vi "autonomous.vi"() -> ()   [LabVIEW 2012, in "Test.lvrbt"]
uses:
  Test.lvrbt
  <vilib>/NXT/Hardware/Plugins/Tetrix DC Motor/TetrixDCMotorAddress.ctl
  <vilib>/NXT/NXTIO Xnodes/NXTIONodeSubVIs/TETRIX IO Check Battery.vi
  <vilib>/NXT/Dual Mode Library/Waits/Wait_Num(msec).vi
  <vilib>/NXT/Dual Mode Library/Waits/Wait_Num.vi
  <vilib>/NXT/NXTIO Xnodes/NXTIONodeSubVIs/TETRIX IO Move DC Motors.vi
  <vilib>/NXT/NXTIO Xnodes/NXTIONodeSubVIs/TETRIX IO Stop DC Motors.vi
  <vilib>/NXT/Subs/LVHSConnector.ctl
  <vilib>/NXT/NXTIO Xnodes/AddressXNode/NXTIOAddress.xnode
  <vilib>/NXT/NXTIO Xnodes/NXTIOXNode/NXTIO.xnode
  <vilib>/NXT/LegoClasses/BrickReference/BrickReference.lvclass
panel:
  out "Enabled":bool
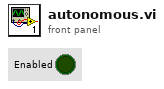
[diagram p1: front panel]
types:
  T1 = typedef "LVHSConnector.ctl" = refnum<class "BrickReference.lvclass">
  T2 = typedef "TetrixDCMotorAddress.ctl" = i32
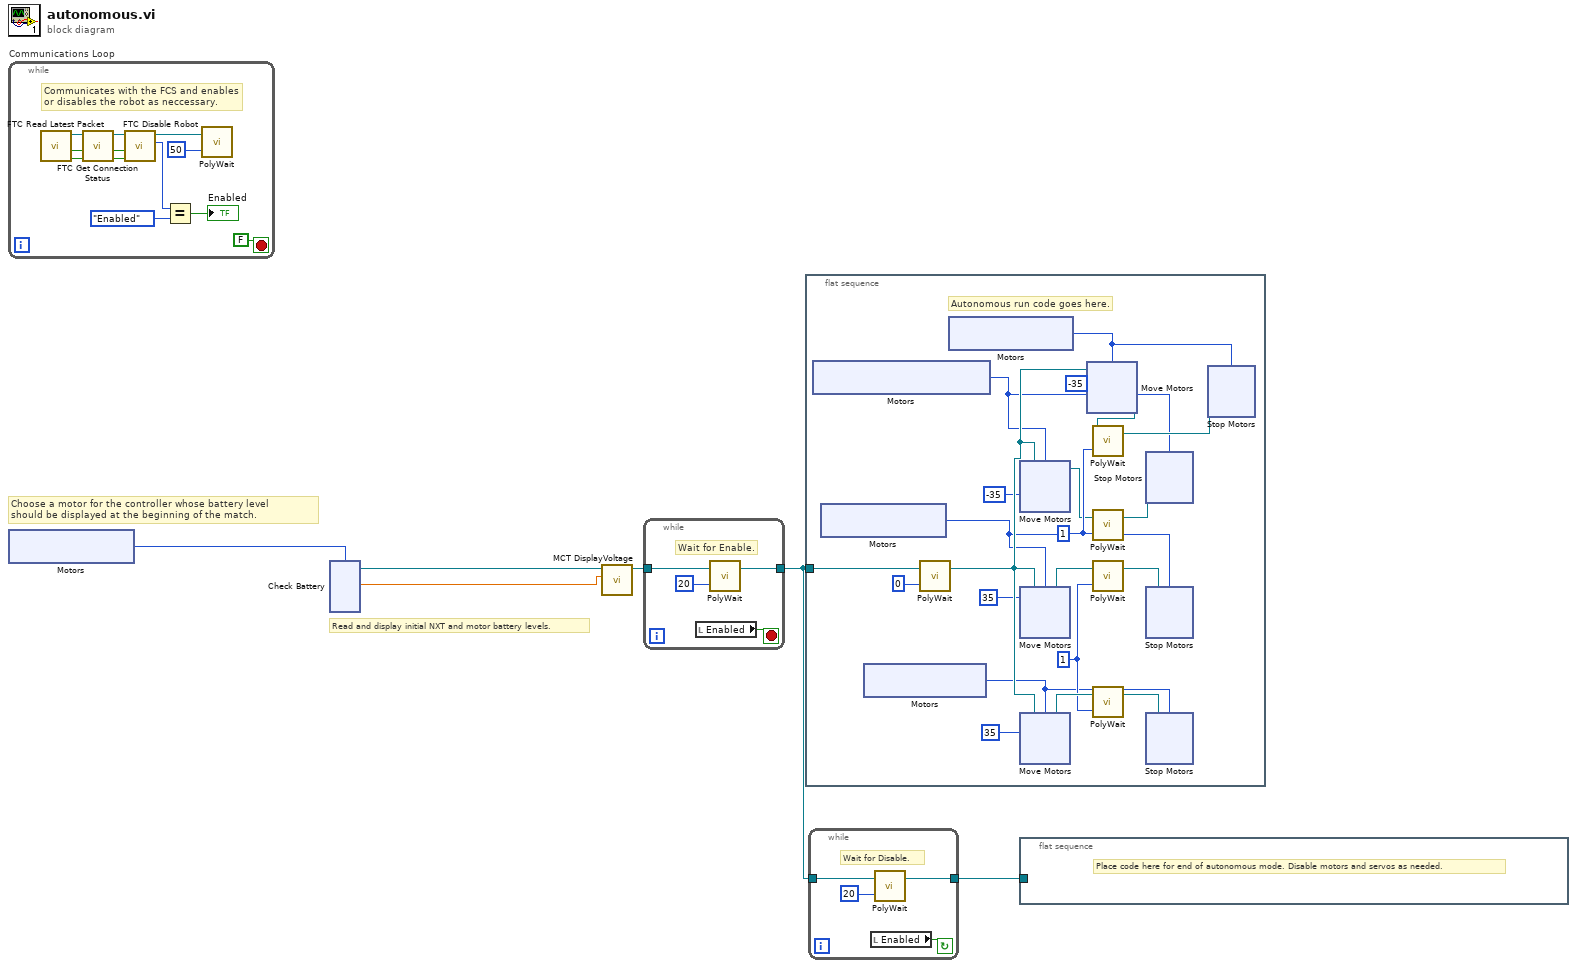
[diagram p0: block diagram]
diagram:
  # "Read and display initial NXT and motor battery levels."
  # "Choose a motor for the controller whose battery level \nshould be displayed at the beginning of the match."
  n1 = while "Communications Loop" {
    stop <- FALSE stop-if-true
    # "Communicates with the FCS and enables \nor disables the robot as neccessary."
    n2 = call <vilib>:"FTC Read Latest Packet.vi"() -> ("Packet Received?"=w16:bool, "Stopped?"=w15:bool, "NXT/EV3"=w18:T1)  [unwired: 6 in, 3 out]
    n3 = call <vilib>:"FTC Get Connection Status.vi"("Packet Received?"=w16, "Stopped?"=w15, "NXT/EV3"=w18) -> ("Online?"=w7:bool, "Stopped?"=w8:bool, "NXT/EV3"=w17:T1)  [unwired: 5 in]
    n4 = call <vilib>:"FTC Disable Robot.vi"("Online?"=w7, "Stopped?"=w8, "NXT/EV3"=w17) -> ("Enabled?"=w11:enum16{"Disabled", "Enabled"}, "NXT/EV3"=w13:T1)  [unwired: 3 in]
    n5 = Equal?(x=w11, y=enum16{"Disabled", "Enabled"}."Enabled") -> (x = y?=→"Enabled":bool)
    n6 = call-poly <vilib>:"PolyWait.vi"("Time (100 msec)"=u32 50 ("Time (msec)"), "NXT/EV3"=w13) -> ()  [unwired: 2 in, 1 out]
  }
  n7 = xnode "Motors"() -> ("Motor"=w1:T2)
  n8 = xnode "Check Battery"("Motors"=w1) -> ("Voltage 1"=w2:sgl, "NXT/EV3"=w4:T1)  [unwired: 1 in]
  n9 = call <vilib>:"MCT DisplayVoltage.vi"("Motor Voltage"=w2, "NXT/EV3"=w4) -> ("NXT/EV3"=w3:T1)  [unwired: 9 in]
  n10 = while {
    tunnel: [w20] -> w6
    tunnel: w3 -> [w19]
    stop <- w21 stop-if-true
    # "Wait for Enable."
    n11 = local read "Enabled"() -> (w21:bool)
    n12 = call-poly <vilib>:"PolyWait.vi"("Time (100 msec)"=u32 20 ("Time (msec)"), "NXT/EV3"=w19) -> ("NXT/EV3"=w20:T1)  [unwired: 2 in]
  }
  n13 = flat-sequence {
    tunnel: w6 -> [w42]
    frame #0 {
      w36 = 1
      w37 = 1
      # "Autonomous run code goes here."
      n14 = xnode "Motors"() -> ("Motor"=w29:T2)
      n15 = xnode ("Motors")() -> ("Motor"=w28:T2)
      n16 = xnode "Motors"() -> ("Motor"=w27:T2)
      n17 = call-poly <vilib>:"PolyWait.vi"("Time (1 sec)"=0, "NXT/EV3"=w42) -> ("NXT/EV3"=w31:T1)  [unwired: 2 in]
      n18 = xnode "Motors"() -> ("Motor"=w30:T2)
      n19 = xnode "Move Motors"("Power/Speed 1"=-35, "Motors"=w29, "NXT/EV3"=w31) -> ("NXT/EV3"=w35:T1)
      n20 = xnode ("Move Motors")("Power/Speed 1"=35, "Motors"=w28, "NXT/EV3"=w31) -> ("NXT/EV3"=w41:T1)
      n21 = xnode "Move Motors"("Power/Speed 1"=35, "Motors"=w27, "NXT/EV3"=w31) -> ("NXT/EV3"=w40:T1)
      n22 = xnode "Move Motors"("Power/Speed 1"=-35, "Motors"=w30, "NXT/EV3"=w31) -> ("NXT/EV3"=w32:T1)
      n23 = call-poly <vilib>:"PolyWait.vi"("Time (1 sec)"=w37, "NXT/EV3"=w32) -> ("NXT/EV3"=w33:T1)  [unwired: 2 in]
      n24 = call-poly <vilib>:"PolyWait.vi"("Time (1 sec)"=w37, "NXT/EV3"=w35) -> ("NXT/EV3"=w34:T1)  [unwired: 2 in]
      n25 = call-poly <vilib>:"PolyWait.vi"("Time (1 sec)"=w36, "NXT/EV3"=w41) -> ("NXT/EV3"=w38:T1)  [unwired: 2 in]
      n26 = call-poly <vilib>:"PolyWait.vi"("Time (1 sec)"=w36, "NXT/EV3"=w40) -> ("NXT/EV3"=w39:T1)  [unwired: 2 in]
      n27 = xnode "Stop Motors"("Motors"=w29, "NXT/EV3"=w34) -> ()  [unwired: 1 out]
      n28 = xnode "Stop Motors"("Motors"=w28, "NXT/EV3"=w38) -> ()  [unwired: 1 out]
      n29 = xnode "Stop Motors"("Motors"=w27, "NXT/EV3"=w39) -> ()  [unwired: 1 out]
      n30 = xnode "Stop Motors"("Motors"=w30, "NXT/EV3"=w33) -> ()  [unwired: 1 out]
    }
  }
  n31 = while {
    tunnel: [w97] -> w5
    tunnel: w6 -> [w96]
    stop <- w98 continue-if-true
    # "Wait for Disable."
    n32 = local read "Enabled"() -> (w98:bool)
    n33 = call-poly <vilib>:"PolyWait.vi"("Time (100 msec)"=u32 20 ("Time (msec)"), "NXT/EV3"=w96) -> ("NXT/EV3"=w97:T1)  [unwired: 2 in]
  }
  n34 = flat-sequence {
    tunnel: w5 -> [_]
    frame #0 {
      # "Place code here for end of autonomous mode. Disable motors and servos as needed."
    }
  }
